vi "Camber controller May 17 2016.vi"() -> ()   [LabVIEW 2014]
uses:
  <vilib>/Instr/_visa.llb/VISA Configure Serial Port (Instr).vi
  Environmental Chamber LabVIEW and Instruments/Drivers and Software/Keithley 2100 Series/Public/Configure/Configure 2 Wire Resistance.vi
  <vilib>/Utility/file.llb/Write To Spreadsheet File (string).vi
  <vilib>/Utility/file.llb/Read From Spreadsheet File (string).vi
  Environmental Chamber LabVIEW and Instruments/Drivers and Software/keithley_6430/Keithley 6430/Public/Data/Read (Single Point).vi
  Environmental Chamber LabVIEW and Instruments/Drivers and Software/LabVIEW 8.2 Drivers/keithley_24xx/Keithley 24XX/Public/Data/Read (Single Point).vi
  Environmental Chamber LabVIEW and Instruments/Drivers and Software/keithley_24xx/Keithley 24XX/Keithley 24XX.lvlib
  Environmental Chamber LabVIEW and Instruments/Drivers and Software/keithley_6430/Keithley 6430/Keithley 6430.lvlib
  Environmental Chamber LabVIEW and Instruments/Drivers and Software/Keithley 2100 Series/Keithley 2100 Series.lvlib
panel:
  out "J-KEM temp chart":dbl(graph)
  out "Elapsed time (min)":dbl
  out "State date/time":string caption="Start time"
  out "Temp (C)":dbl
  in  "Tare elapsed time":bool
  in  "Stop program when sequence ends":bool=TRUE
  out "K-2100 (Ohm)":cluster{"Measurement":dbl}(graph)
  out "pressure chart":cluster{"pressure":dbl}(graph)
  out "K-6430 (Ohm)":cluster{"Measurement":dbl}(graph)
  out "K-2420 (Ohm)":cluster{"Resistance":sgl}(graph)
  in  "Data saving options":T1={"Save during sequence only"=TRUE, "Save now"=FALSE, "Delay between data points (s)"=0.0, "Experiment Notes"="", "Currently saving data"=FALSE, "Data file save path"=path ""} {"Delay between data points (s)" min=0.0 max=30.0 format="%#_13g"}
  in  "Set pressure parameters":T2={"valve % open"=100.0, "Desired pressure"=0.0, "Vapor sccm"=0.0, "Gas sccm"=0.0, "Valve"=enum."% Open", "Pressure Mode"=enum."Abs. pressure", "analyte partial pressure"=100.0} {"analyte partial pressure" min=0.0 max=100.0 step=5.0; "Gas sccm" min=0 max=200 step=5; "Vapor sccm" min=0 max=200 step=5; "Desired pressure" min=0.0 max=760.0 step=5.0; "valve % open" min=0.0 max=100.0 step=5.0 format="%#_2f"}
  out "Actual":T3 {"actual gas flow" format="%#_3g"; "Actual vapor flow" format="%#_3g"; "actual pressure" format="%#_3g"; "Valve position (%)" format="%#_2f"}
  out "Arduino QCM freq":T4 {"QCM1" format="%#_8g"; "QCM2" format="%#_8g"; "QCM3" format="%#_8g"; "QCM4" format="%#_8g"; "QCM5" format="%#_8g"}
  out "Arduino QCM plots":T5
  in  "Sample names":T6={"QCM1"="aQCM2", "QCM2"="aQCM2", "QCM3"="aQCM3", "QCM4"="aQCM4", "QCM5"="aQCM5", "QCM6"="aQCM6", "SRS"="sample_SRS", "K-2420"="Keithley2420", "K-6430"="Keithley6430", "K-2100"="Keithley6430"}
  out "Sequence\npreview":cluster{dbl[], dbl[]}[](graph)
  in  "Gate time":u16(ring)=1 items=["0.1 seconds", "1.0 seconds", "10.0 seconds"]
  out "MHz":dbl format="%.8f"
  out "QCM plot":T7(graph)
  in  "User-defined\nsequence":string[][](table) caption="Create sequence"
  out "Sequence end time":string
  in  "Run Sequence":bool
  in  "Import sequence file":bool
  in  "Save sequence":bool
  in  "Clear sequence":bool
  in  "Turbo pump\nauto on":bool=TRUE caption="Turbo pump auto on"
  in  "Stop":bool
  in  "Clear all charts":bool
  out "appended array":dbl[](array[numeric]) caption="atm\nTorr"
  in  "rapidox O2 Sensor":bool
  in  "setnag O2 Pump":bool
  in  "Baud Rate 2":i32(ring)=2 items=["2400", "4800", "9600", "19200", "38400", "57600", "115200"]
  in  "Com Port":i32(ring) items=["Com 1", "Com 2", "Com 3", "Com 4", "Com 5", "Com 6", "COM 7", "COM 8", "COM 9", "COM 10", "COM 11", "COM 12", "com 13", "COM 14"]
  in  "Com Port 2":i32(ring) items=["Com 1", "Com 2", "Com 3", "Com 4", "Com 5", "Com 6", "COM 7", "COM 8", "COM 9", "COM 10", "COM 11", "COM 12", "com 13", "COM 14"]
  out "Waveform Chart":cluster{dbl}(graph)
  out "O2 Concentration (PPM)":dbl
  out "Waveform Chart 6":cluster{dbl}(graph)
  # "Pressure Control"
  # "Gas Sequence"
  # "SRS QCM"
  # "Currently Unused"
  # "100%"
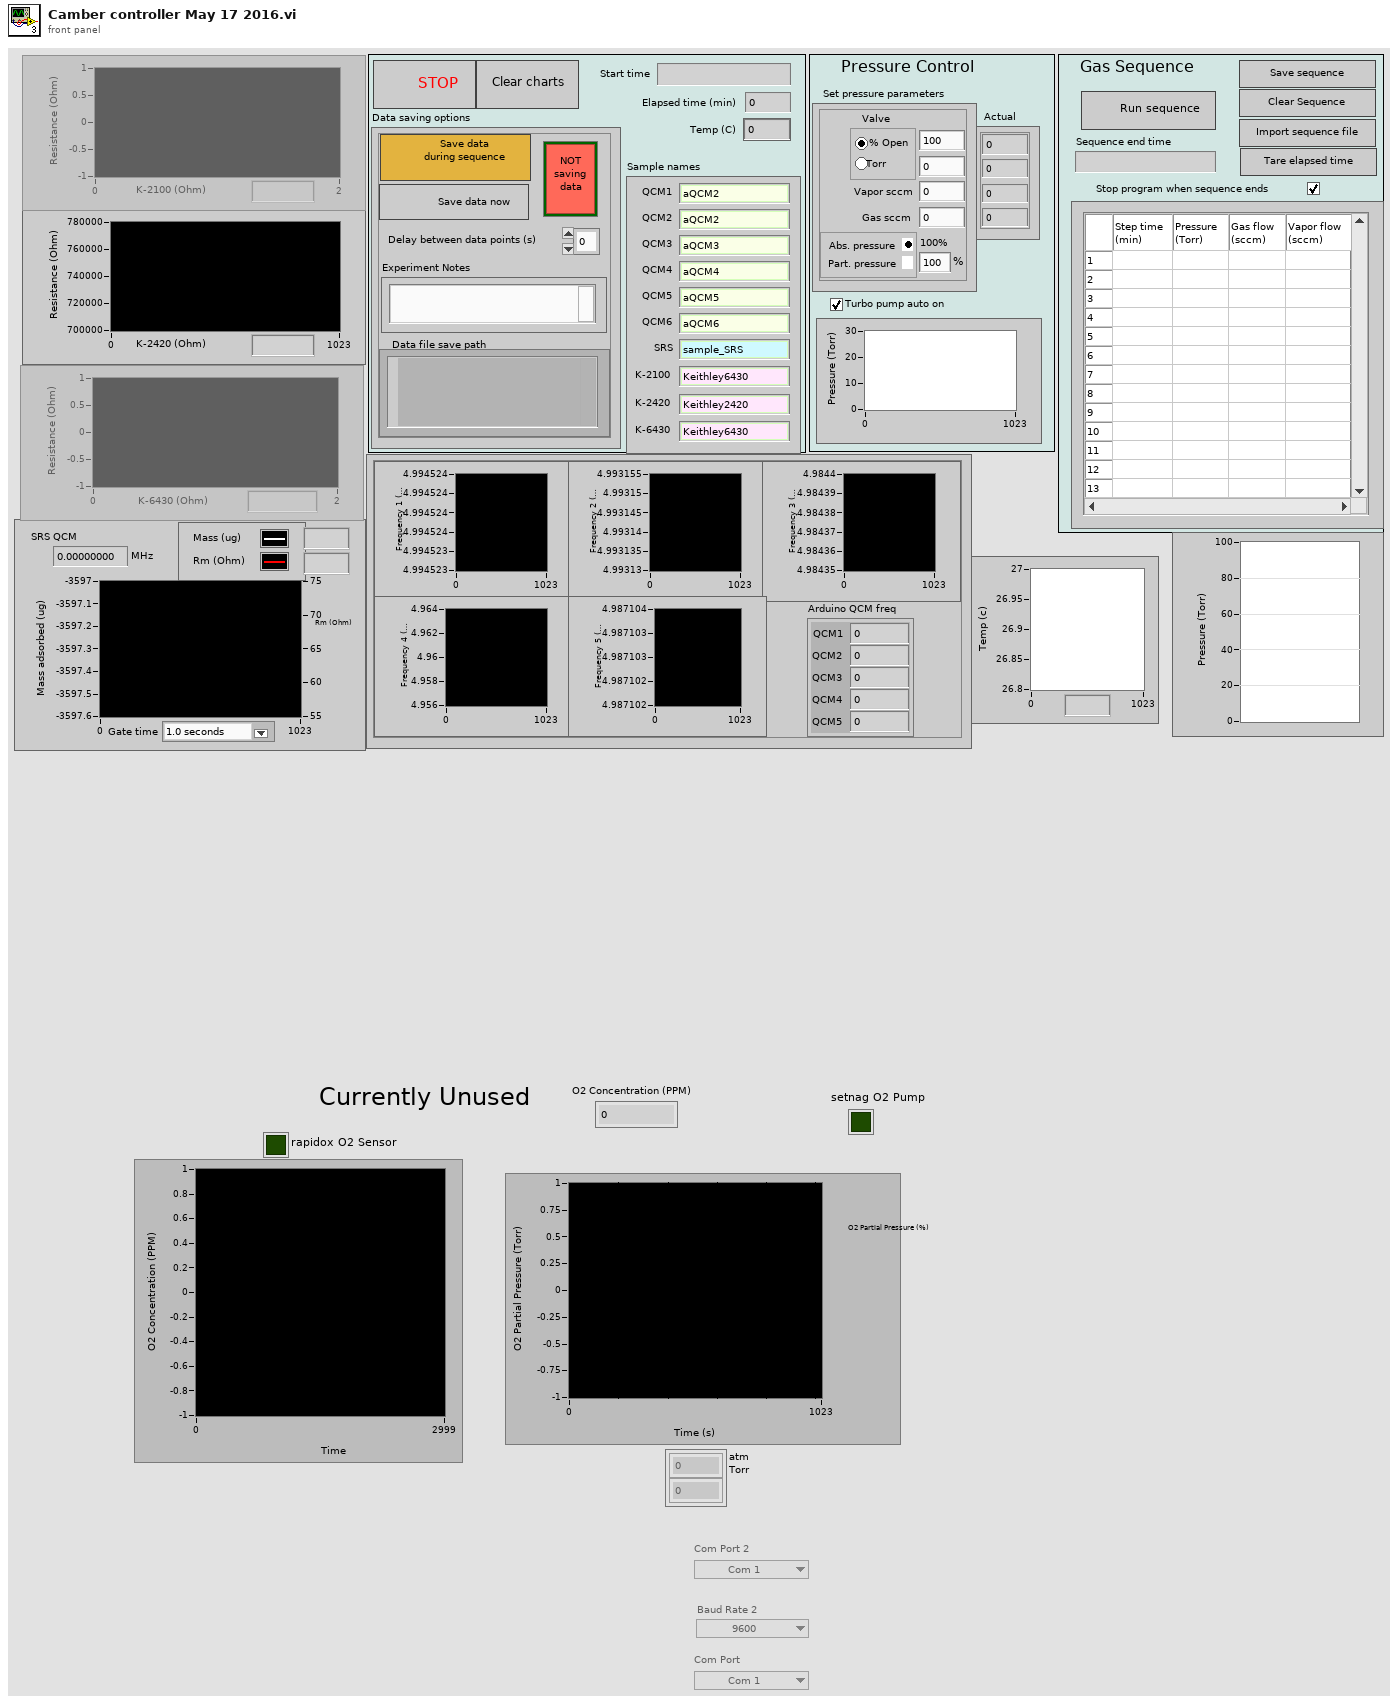
[diagram p1: front panel]
types:
  T1 = cluster{"Save during sequence only":bool, "Save now":bool, "Delay between data points (s)":dbl, "Experiment Notes":string, "Currently saving data":bool, "Data file save path":path}
  T2 = cluster{"valve % open":dbl, "Desired pressure":dbl, "Vapor sccm":sgl, "Gas sccm":sgl, "Valve":enum32{"% Open", "Torr "}, "Pressure Mode":enum32{"Abs. pressure", " Part. pressure"}, "analyte partial pressure":dbl}
  T3 = cluster{"Valve position (%)":dbl, "actual pressure":dbl, "Actual vapor flow":dbl, "actual gas flow":dbl}
  T4 = cluster{"QCM1":dbl, "QCM2":dbl, "QCM3":dbl, "QCM4":dbl, "QCM5":dbl}
  T5 = cluster{"arduino qcm 1":dbl, "arduino qcm 2":dbl, "arduino qcm 3":dbl, "arduino qcm 4":dbl, "arduino qcm 5":dbl}
  T6 = cluster{"QCM1":string, "QCM2":string, "QCM3":string, "QCM4":string, "QCM5":string, "QCM6":string, "SRS":string, "K-2420":string, "K-6430":string, "K-2100":string}
  T7 = cluster{"Numeric Control":dbl, "Resistance out":dbl}
  T8 = cluster{"Arduino 1":refnum<visa-resource-name>, "Arduino 2":refnum<visa-resource-name>, "Arduino 3":refnum<visa-resource-name>, "Arduino 4":refnum<visa-resource-name>, "Arduino 5":refnum<visa-resource-name>}
  T9 = enum16{"open", "open or create", "create or replace", "create", "open (read only)"}
  T10 = enum8{"Enabled", "Disabled", "Disabled and Grayed Out"}
  T11 = enum16{"no parity", "odd parity", "even parity", "mark parity", "space parity"}
  T12 = cluster{"task out":refnum<k21>, "error out":errorcluster, "task out":refnum<k21>, "error out":errorcluster, "task out":refnum<k21>, "error out":errorcluster, "VISA resource name":refnum<visa-resource-name>, "error out":errorcluster}
  T13 = cluster{"task out":refnum<k21>, "error out":errorcluster, "task out":refnum<k21>, "error out":errorcluster, "task out":refnum<k21>, "error out":errorcluster, "VISA resource name out":refnum<visa-resource-name>, "error out":errorcluster}
  T14 = cluster{bool, "VISA resource name":refnum<visa-resource-name>, "error out":errorcluster}
  T15 = cluster{bool, "VISA resource name out":refnum<visa-resource-name>, "error out":errorcluster}
  T16 = cluster{"VISA resource name out":refnum<visa-resource-name>, "error out":errorcluster, "VISA resource name out":refnum<visa-resource-name>, "error out":errorcluster, "VISA resource name out":refnum<visa-resource-name>, "error out":errorcluster, "VISA resource name out":refnum<visa-resource-name>, "error out":errorcluster, "VISA resource name out":refnum<visa-resource-name>, "error out":errorcluster}
  T17 = cluster{"f":dbl, "f":dbl, "f":dbl, "f":dbl, "f":dbl}
  T18 = cluster{"String":string, "String":string, "String":string}
  T19 = cluster{"Boolean":bool, "VISA resource name out":refnum<visa-resource-name>, "error out":errorcluster}
  T20 = cluster{bool, "VISA out":refnum<visa-resource-name>, "error out":errorcluster}
  T21 = cluster{"Boolean":bool, "VISA out":refnum<visa-resource-name>, "error out":errorcluster}
  T22 = cluster{"Numeric Control":dbl, "Cluster":cluster{"Numeric Control":dbl}, "String":string, "error out":errorcluster}
  T23 = cluster{bool, "Com Port":i32, "Numeric Control out":dbl}
  T24 = cluster{"String data out":string, string, string, string}
  T25 = cluster{"User-defined\nsequence":refnum<vi>, "Sequence end time":refnum<vi>, "Run Sequence":refnum<vi>}
  T26 = cluster{"Present (s)":dbl, "Run Sequence":bool, "Set pressure parameters":cluster{"valve % open":dbl, "Desired pressure":dbl, "Vapor sccm":sgl, "Gas sccm":sgl, "Valve":enum32{"% Open", "Torr "}, "Pressure Mode":enum32{"Abs. pressure", " Part. pressure"}, "analyte partial pressure":dbl}, "sequence end time":timestamp}
  T27 = cluster{bool, "Turbo pump\nauto on":bool, "current  step # out":i32, cluster{"Present (s)":dbl, "Run Sequence":bool, "Set pressure parameters":cluster{"valve % open":dbl, "Desired pressure":dbl, "Vapor sccm":sgl, "Gas sccm":sgl, "Valve":enum32{"% Open", "Torr "}, "Pressure Mode":enum32{"Abs. pressure", " Part. pressure"}, "analyte partial pressure":dbl}, "sequence end time":timestamp}}
  T28 = cluster{"pressure":string, "RH":string, "gas flow":string, "vapor flow":string}
  T29 = cluster{"Valve position (%)":dbl, "pressure":dbl, "vapor flow":dbl, "gas flow":dbl}
  T30 = cluster{"sequence on?":bool, "current  step # out":i32, "sequence end time":timestamp}
  T31 = cluster{"task out":refnum<k21>, "error out":errorcluster, "task out":refnum<k21>, "error out":errorcluster, "task out":refnum<k21>, "error out":errorcluster, "VISA Refnum out":refnum<visa-resource-name>, "error out":errorcluster}
  T32 = cluster{"VISA Refnum out":refnum<visa-resource-name>, "error out":errorcluster, "VISA Refnum out":refnum<visa-resource-name>, "error out":errorcluster, "VISA Refnum out":refnum<visa-resource-name>, "error out":errorcluster, "VISA Refnum out":refnum<visa-resource-name>, "error out":errorcluster, "VISA Refnum out":refnum<visa-resource-name>, "error out":errorcluster}
  T33 = cluster{"f":string, "f":string, "f":string, "f":string, "f":string}
  T34 = cluster{"f":dbl, "f":dbl, "f":dbl, "f":dbl, "f":dbl}[]
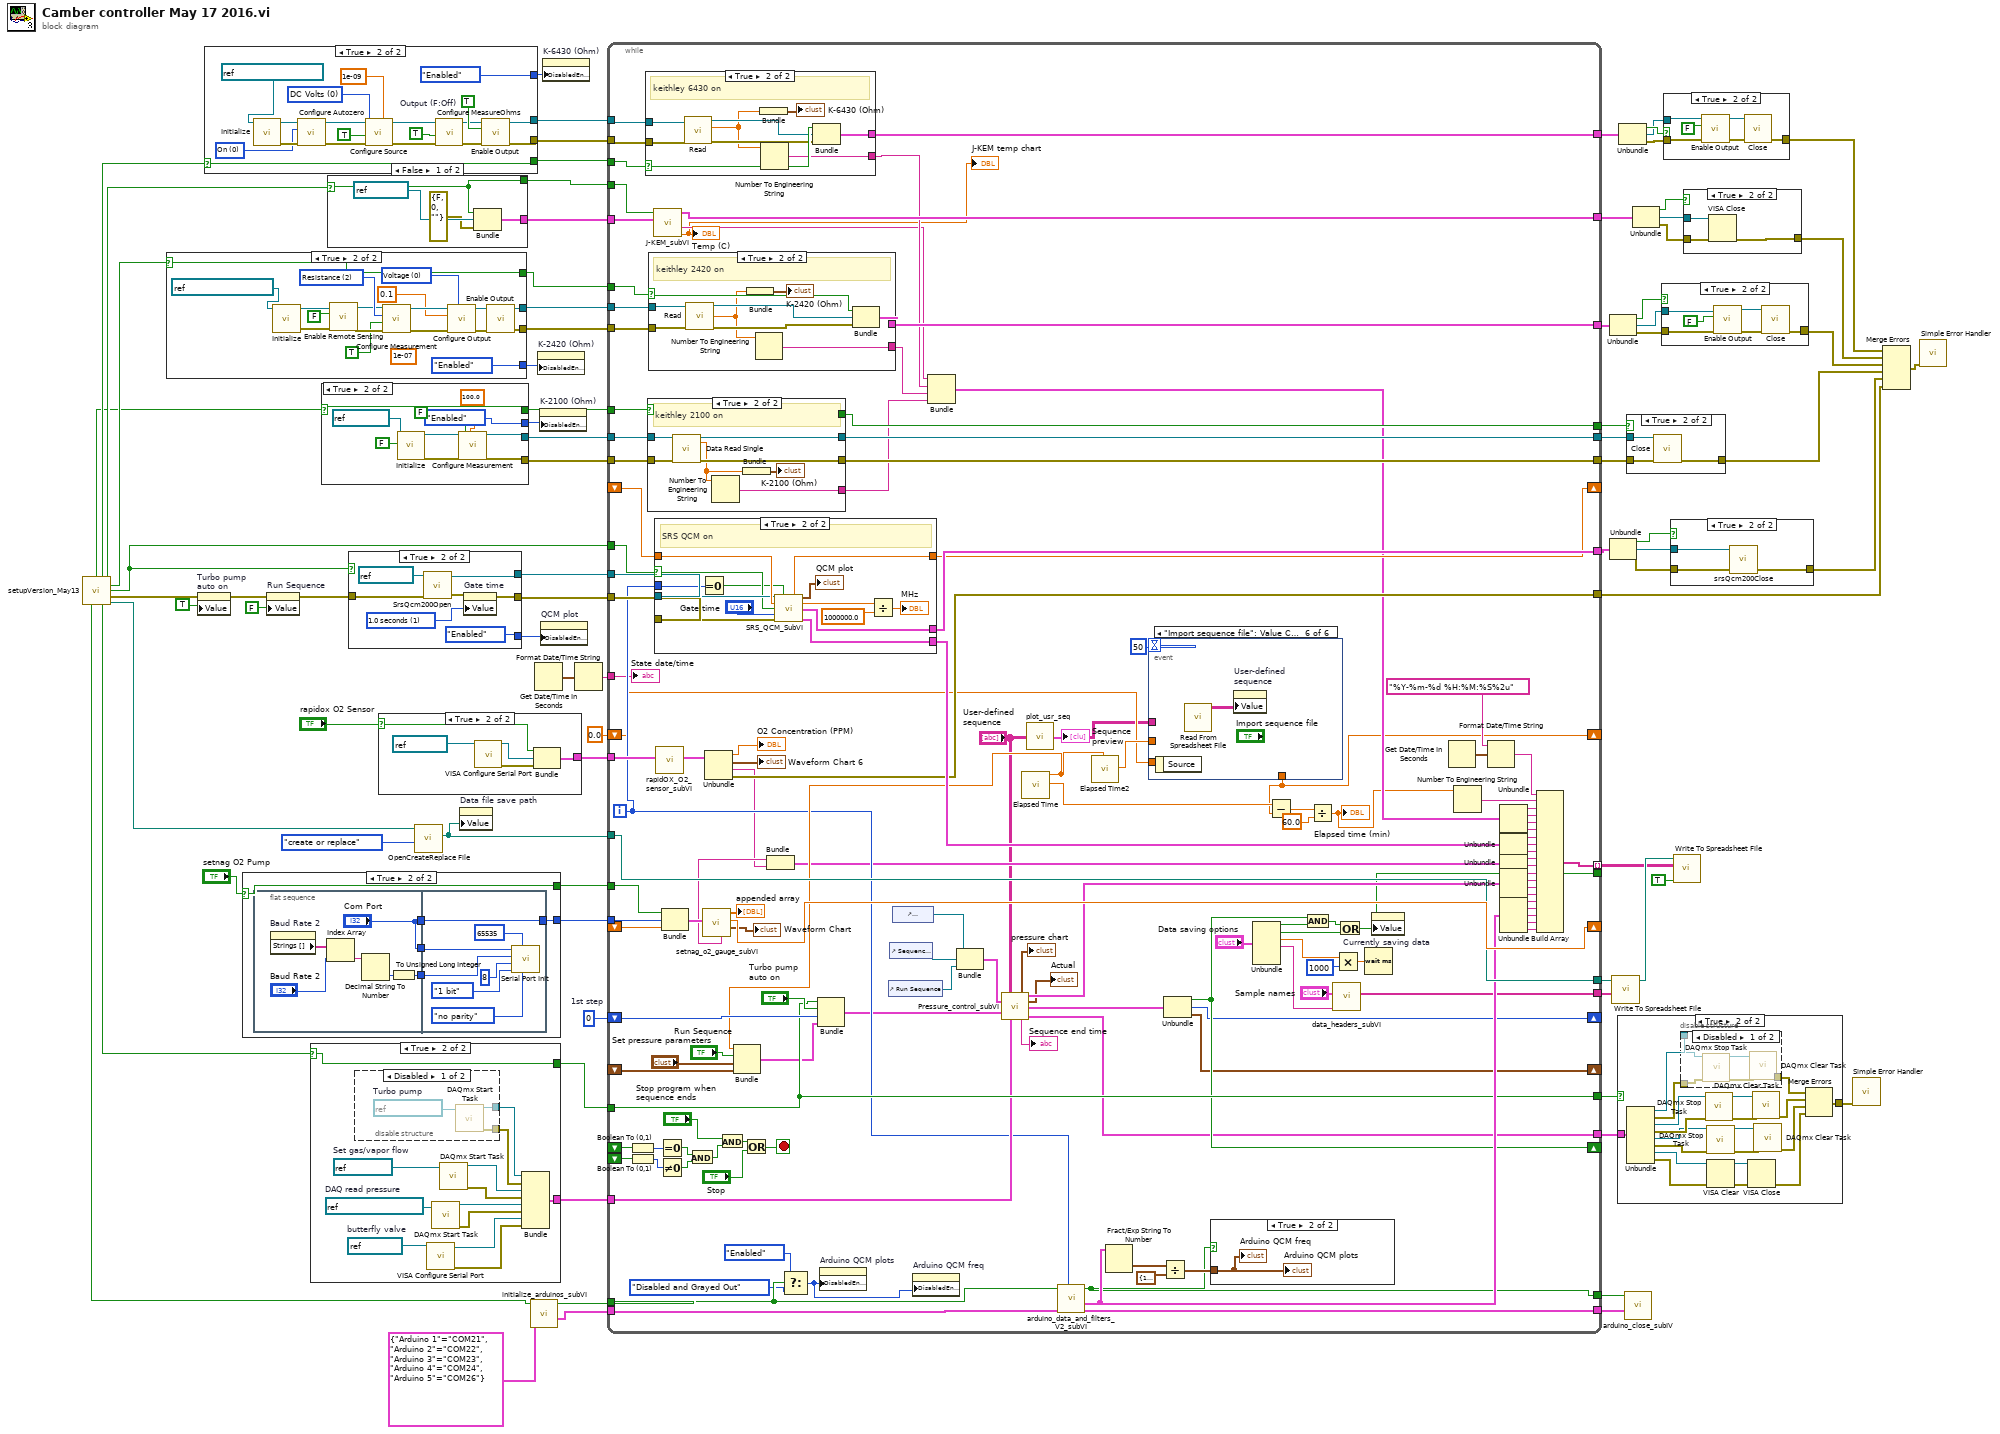
[diagram p0: block diagram]
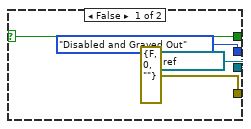
[diagram p3: hidden frame]
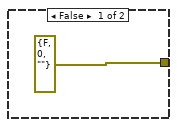
[diagram p4: hidden frame]
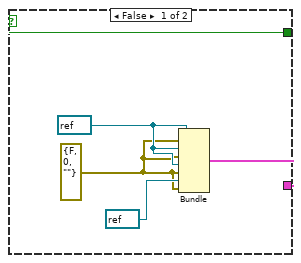
[diagram p6: hidden frame]
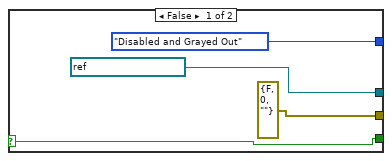
[diagram p9: hidden frame]
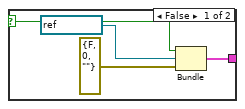
[diagram p10: hidden frame]
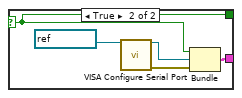
[diagram p12: hidden frame]
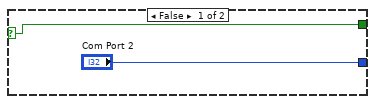
[diagram p13: hidden frame]
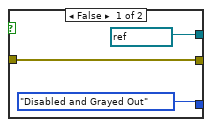
[diagram p15: hidden frame]
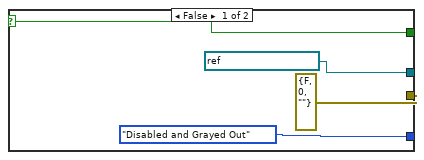
[diagram p17: hidden frame]
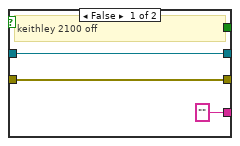
[diagram p19: hidden frame]
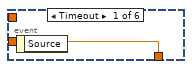
[diagram p20: hidden frame]
diagram:
  w42 = 0  # 1st step
  n1 = call "setupVersion_May13.vi"() -> ("Keithley 2100 out"=w11:bool, "Keithley 6431"=w35:bool, "J-KEM2"=w34:bool, "Keithley 2421"=w23:bool, "SRS QCM 2"=w37:bool, "error IO"=w1:errorcluster, "Arduino2"=w28:bool, "Pressure control 2"=w36:bool, "Save file path 2"=w2:path)  [unwired: 7 in]
  n2 = case shown="True" w23 {
    selector: w23 -> [w83 w87]
    tunnel: [refnum<visa-resource-name> "GPIB1::24::INSTR" ("VISA resource name") w96] -> w80
    tunnel: [errorcluster {"status"=FALSE, "code"=0, "source"=""} ("error out") w91] -> w79
    tunnel: [T10."Disabled and Grayed Out" ("Disabled") T10."Enabled" ("Disabled")] -> w32
    tunnel: [w83 w87] -> w22
    frame False {
    }
    frame True {
      (unwired) 1e-07 ("Manual Range (1.0)")
      w98 = u16 0 items=["Voltage", "Current"] ("Source Mode  (0: Voltage)")
      w103 = u16 2 items=["Volts", "Current", "Resistance"] ("Function (0: Volts)")
      n3 = call "Initialize.vi"("VISA resource name"=refnum<visa-resource-name> "GPIB1::24::INSTR") -> ("error out"=w92:errorcluster, "VISA resource name out"=w95:refnum<visa-resource-name>)  [unwired: 9 in]
      n4 = call "Enable Remote Sensing.vi"("error in (no error)"=w92, "Enable Remote Sensing (T: Enable)"=FALSE ("4-wire?"), "VISA resource name"=w95) -> ("error out"=w93:errorcluster, "VISA resource name out"=w94:refnum<visa-resource-name>)  [unwired: 7 in]
      n5 = call "Configure Measurement.vi"("error in (no error)"=w93, "Enable Auto Range (T:Enable)"=TRUE, "Function (0: Volts)"=w103, "VISA resource name"=w94) -> ("error out"=w102:errorcluster, "VISA resource name out"=w101:refnum<visa-resource-name>)  [unwired: 6 in]
      n6 = call "Configure Output.vi"("Source Mode  (0: Voltage)"=w98, "error in (no error)"=w102, "Output Level (0)"=0.1 ("Applied Voltage (V)"), "VISA resource name"=w101) -> ("error out"=w100:errorcluster, "VISA resource name out"=w99:refnum<visa-resource-name>)  [unwired: 6 in]
      n7 = call "Enable Output.vi"("error in (no error)"=w100, "VISA resource name"=w99) -> ("error out"=w91:errorcluster, "VISA resource name out"=w96:refnum<visa-resource-name>)  [unwired: 8 in]
    }
  }
  n8 = property on="Turbo pump\nauto on" class="Bool (strict)"(error in=w1, "Value"=TRUE ("Turbo\npump")) -> (error out=w38:errorcluster)  [unwired: 1 in, 1 out]
  n9 = case shown="True" w35 {
    selector: w35 -> [w105 w109]
    tunnel: [refnum<visa-resource-name> "GPIB0::29::INSTR" ("VISA resource name") w122] -> w49
    tunnel: [errorcluster {"status"=FALSE, "code"=0, "source"=""} ("error out") w123] -> w48
    tunnel: [T10."Disabled and Grayed Out" ("Disabled") T10."Enabled" ("Disabled")] -> w31
    tunnel: [w105 w109] -> w21
    frame False {
    }
    frame True {
      w111 = u16 0 items=["DC Volts", "DC Current"] ("Source Function (0: DC Volts)")
      w118 = u16 0 items=["On", "Off", "Once"] ("Autozero  (0: On)")
      w126 = TRUE  # Output (F:Off)
      n10 = call "Initialize.vi"("VISA resource name"=refnum<visa-resource-name> "GPIB0::30::INSTR") -> ("error out"=w119:errorcluster, "VISA resource name out"=w120:refnum<visa-resource-name>)  [unwired: 4 in, 5 out]
      n11 = call "Configure Autozero.vi"("error in (no error)"=w119, "Autozero  (0: On)"=w118, "VISA resource name"=w120) -> ("error out"=w114:errorcluster, "VISA resource name out"=w116:refnum<visa-resource-name>)  [unwired: 7 in]
      n12 = call "Configure Source.vi"("I-Source Level [A]"=1e-09, "error in (no error)"=w114, "Auto Range (T:Enable)"=TRUE, "Source Function (0: DC Volts)"=w111, "VISA resource name"=w116) -> ("error out"=w113:errorcluster, "VISA resource name out"=w115:refnum<visa-resource-name>)  [unwired: 5 in]
      n13 = call "Configure MeasureOhms.vi"("error in (no error)"=w113, "Auto Range (T:Enable)"=TRUE, "VISA resource name"=w115) -> ("error out"=w127:errorcluster, "VISA resource name out"=w125:refnum<visa-resource-name>)  [unwired: 3 in, 4 out]
      n14 = call "Enable Output.vi"("error in (no error)"=w127, "Enable Output (F:Off)"=w126, "VISA resource name"=w125) -> ("error out"=w123:errorcluster, "VISA resource name out"=w122:refnum<visa-resource-name>)  [unwired: 7 out]
    }
  }
  n15 = case shown="True" "setnag O2 Pump" {
    selector: "setnag O2 Pump" -> [w128 w130]
    tunnel: ["Com Port 2" w131] -> w76
    tunnel: [w128 w130] -> w8
    frame False {
    }
    frame True {
      n16 = flat-sequence {
        tunnel: ["Com Port"] -> w134
        tunnel: [w136] -> w133
        tunnel: ["Com Port"] -> w132
        tunnel: w134 -> [w142]
        tunnel: w133 -> [w141]
        tunnel: w132 -> [w143]
        tunnel: [w143] -> w131
        frame #0 {
          n17 = property on="Baud Rate 2" class="Ring (strict)"() -> ("Strings []"=w138:string[])  [unwired: 2 in, 2 out]
          n18 = Index Array(array=w138, index="Baud Rate 2") -> (element=w139:string)
          n19 = Decimal String To Number(string=w139) -> (number=w137:i32)  [unwired: 2 in, 1 out]
          n20 = To Unsigned Long Integer(number=w137) -> (unsigned 32bit integer=w136:u32)
        }
        frame #1 {
          n21 = call <vilib>:"Serial Port Init.vi"("parity"=T11."no parity", "buffer size"=u16 65535, "stop bits"=enum16{"1 bit", "1.5 bits", "2 bits"}."1 bit", "data bits"=u16 8, "baud rate"=w141, "port number"=w142) -> ()  [unwired: 1 in, 1 out]
        }
      }
    }
  }
  n22 = property on="Run Sequence" class="Bool (strict)"(error in=w38, "Value"=FALSE ("Run Sequence")) -> (error out=w40:errorcluster)  [unwired: 1 in, 1 out]
  n23 = case shown="True" w36 {
    selector: w36 -> [w148 w153]
    tunnel: [w149 w155] -> w43
    tunnel: [w148 w153] -> w20
    frame False {
      w151 = refnum<k21> refnum ("task out")
      w150 = errorcluster {"status"=FALSE, "code"=0, "source"=""} ("error out")
      n24 = Bundle("task out"=w151, "error out"=w150, "task out"=w151, "error out"=w150, "task out"=w151, "error out"=w150, "VISA resource name"=refnum<visa-resource-name> refnum, "error out"=w150) -> (w149:T12)  [unwired: 1 in]
    }
    frame True {
      w163 = refnum<visa-resource-name> "COM5"  # butterfly valve
      w164 = refnum<k21> "Setflow"  # Set gas/vapor flow
      w165 = refnum<k21> "AllDaqReadings"  # DAQ read pressure
      n25 = disable-structure shown="Disabled" {
        disable-tunnel: [w167 _] -> w162
        disable-tunnel: [w166 _] -> w161
        frame Disabled {
          w168 = refnum<k21> "TurboON"  # Turbo pump
          n26 = call <vilib>:"DAQmx Start Task.vi"("task/channels in"=w168) -> ("task out"=w167:refnum<k21>, "error out"=w166:errorcluster)  [unwired: 13 in]
        }
        frame Enabled {
        }
      }
      n27 = call-poly "VISA Configure Serial Port"("VISA resource name"=w163) -> ("VISA resource name out"=w156:refnum<visa-resource-name>, "error out"=w154:errorcluster)  [unwired: 13 in]
      n28 = call <vilib>:"DAQmx Start Task.vi"("task/channels in"=w165) -> ("task out"=w158:refnum<k21>, "error out"=w157:errorcluster)  [unwired: 13 in]
      n29 = call <vilib>:"DAQmx Start Task.vi"("task/channels in"=w164) -> ("task out"=w160:refnum<k21>, "error out"=w159:errorcluster)  [unwired: 13 in]
      n30 = Bundle("task out"=w162, "error out"=w161, "task out"=w160, "error out"=w159, "task out"=w158, "error out"=w157, "VISA resource name out"=w156, "error out"=w154) -> (w155:T13)  [unwired: 1 in]
    }
  }
  n31 = case shown="True" w11 {
    selector: w11 -> [w170 w176]
    tunnel: [refnum<visa-resource-name> "K-2100" ("VISA resource name out") w179] -> w18
    tunnel: [errorcluster {"status"=FALSE, "code"=0, "source"=""} ("error out") w178] -> w17
    tunnel: [w170 w176] -> w16
    tunnel: [T10."Disabled and Grayed Out" ("Disabled") T10."Enabled" ("Disabled")] -> w10
    frame False {
    }
    frame True {
      n32 = call "Initialize.vi"("VISA resource name"=refnum<visa-resource-name> "K-2100", "Reset? (T: Reset)"=FALSE) -> ("VISA resource name out"=w180:refnum<visa-resource-name>, "error out"=w177:errorcluster)  [unwired: 16 in]
      n33 = call-poly "Configure Measurement.vi"("VISA resource name"=w180, "error in (no error)"=w177, "Auto Range? (T: Auto)"=FALSE, "Custom Range (100 Ohm)"=100.0 ("Temp (C) 2")) -> ("VISA resource name out"=w179:refnum<visa-resource-name>, "error out"=w178:errorcluster)  [unwired: 14 in]
    }
  }
  n34 = case shown="False" w34 {
    selector: w34 -> [w183 w188]
    tunnel: [w184 w189] -> w65
    tunnel: [w183 w188] -> w59
    frame False {
      n35 = Bundle(w183, "VISA resource name"=refnum<visa-resource-name> "COM3", "error out"=errorcluster {"status"=FALSE, "code"=0, "source"=""}) -> (w184:T14)  [unwired: 1 in]
    }
    frame True {
      n36 = call-poly "VISA Configure Serial Port"("VISA resource name"=refnum<visa-resource-name> "COM3") -> ("VISA resource name out"=w190:refnum<visa-resource-name>, "error out"=w187:errorcluster)  [unwired: 13 in]
      n37 = Bundle(w188, "VISA resource name out"=w190, "error out"=w187) -> (w189:T15)  [unwired: 1 in]
    }
  }
  n38 = case shown="True" w37 {
    tunnel: [refnum<visa-resource-name> "COM6" ("VISA in") w198] -> w78
    tunnel: [w193 w195] -> w77
    tunnel: w40 -> [w193 w200]
    tunnel: [T10."Disabled and Grayed Out" ("Disabled") T10."Enabled" ("Disabled")] -> w33
    frame False {
    }
    frame True {
      w197 = u16 1 items=["0.1 seconds", "1.0 seconds", "10.0 seconds"] ("Gate time")
      n39 = call "SrsQcm200Open.vi"("error in"=w200, "VISA in"=refnum<visa-resource-name> "COM6") -> ("error out"=w196:errorcluster, "VISA out"=w198:refnum<visa-resource-name>)  [unwired: 3 in]
      n40 = property on="Gate time" class="Ring (strict)"(error in=w196, "Value"=w197) -> (error out=w195:errorcluster)  [unwired: 1 in, 1 out]
    }
  }
  n41 = case shown="True" "rapidox O2 Sensor" {
    selector: "rapidox O2 Sensor" -> [w202 w207]
    tunnel: [w203 w208] -> w55
    frame False {
      n42 = Bundle(w202, "VISA resource name"=refnum<visa-resource-name> "COM7", "error out"=errorcluster {"status"=FALSE, "code"=0, "source"=""}) -> (w203:T14)  [unwired: 1 in]
    }
    frame True {
      n43 = call-poly "VISA Configure Serial Port"("VISA resource name"=refnum<visa-resource-name> "COM7") -> ("VISA resource name out"=w209:refnum<visa-resource-name>, "error out"=w206:errorcluster)  [unwired: 13 in]
      n44 = Bundle(w207, "VISA resource name out"=w209, "error out"=w206) -> (w208:T15)  [unwired: 1 in]
    }
  }
  n45 = call "OpenCreateReplace File.vi"("function (open:0)"=T9."create or replace", "file path"=w2) -> ("new file path"=w19:path)  [unwired: 6 in, 3 out]
  n46 = property on="Data file save path" class="Path"("Value"=w19) -> ()  [unwired: 2 in, 2 out]
  n47 = call "initialize_arduinos_subVI.vi"("arduino 1-6 addresses"=T8 {"Arduino 1"="COM21", "Arduino 2"="COM22", "Arduino 3"="COM23", "Arduino 4"="COM24", "Arduino 5"="COM26"}, "arduinos on?"=w28) -> ("arduino addresses/errors"=w3:T16, "arduinos on/off"=w29:bool)  [unwired: 8 in]
  n48 = Get Date/Time In Seconds() -> (seconds since 1Jan1904=w82:timestamp)
  n49 = property on="K-2420 (Ohm)" class="WFChart (strict)"("DisabledEnum"=w32) -> ()  [unwired: 2 in, 2 out]
  n50 = property on="K-2100 (Ohm)" class="WFChart (strict)"("DisabledEnum"=w10) -> ()  [unwired: 2 in, 2 out]
  n51 = property on="QCM plot" class="WFChart (strict)"("DisabledEnum"=w33) -> ()  [unwired: 2 in, 2 out]
  n52 = property on="K-6430 (Ohm)" class="WFChart (strict)"("DisabledEnum"=w31) -> ()  [unwired: 2 in, 2 out]
  n53 = Format Date/Time String(seconds (now)=w82) -> (date/time string=w7:string)  [unwired: 2 in]
  n54 = while {
    shift-right: [w346] -> _
    shift-left: _ -> [w240]
    tunnel: [w329] -> w30 mode=indexing if=w274
    tunnel: w22 -> [w335]
    tunnel: w80 -> [w345]
    tunnel: w79 -> [w344]
    tunnel: w78 -> [w343]
    tunnel: w77 -> [w342]
    tunnel: w37 -> [w341]
    tunnel: w8 -> [w242]
    tunnel: w76 -> [w243]
    tunnel: [w340] -> w73
    tunnel: [w339] -> w69
    tunnel: w65 -> [w338]
    tunnel: [w337] -> w64
    tunnel: w59 -> [w336]
    tunnel: w55 -> [w257]
    tunnel: [w253] -> w5
    tunnel: [w334] -> w54
    tunnel: w19 -> [w334]
    shift-right: [w327] -> _
    shift-left: _ -> [w328]
    tunnel: w49 -> [w333]
    tunnel: w48 -> [w332]
    tunnel: [w331] -> w47
    tunnel: w20 -> [w292]
    tunnel: [w292] -> w44
    tunnel: w43 -> [w290]
    shift-right: [w215] -> _
    shift-left: w42 -> [w294]
    tunnel: [w274] -> _
    shift-right: [w214] -> _
    shift-left: _ -> [w302]
    tunnel: w29 -> [w252]
    tunnel: w3 -> [w320]
    tunnel: [w248] -> w26
    tunnel: [w319] -> w27
    tunnel: [w311] -> w25
    tunnel: [w213] -> w24
    tunnel: w21 -> [w303]
    shift-right: [w216] -> _
    shift-left: _ -> [w289]
    shift-left: _ -> [w288]
    tunnel: w18 -> [w272]
    tunnel: w17 -> [w271]
    tunnel: w16 -> [w270]
    tunnel: [w269] -> w15
    tunnel: [w268] -> w14
    tunnel: [w267] -> w13
    shift-right: [w234] -> _
    shift-left: 0.0 ("Elapsed Time (s)") -> [w235]
    tunnel: w7 -> [w225]
    i -> [w244]
    stop <- w278 stop-if-true
    n55 = Boolean To (0,1)(Boolean=w289) -> (0, 1=w287:i16)
    n56 = Boolean To (0,1)(Boolean=w288) -> (0, 1=w286:i16)
    n57 = case "Keithley 6430" shown="True" w303 {
      selector: w303 -> [w376 w386]
      tunnel: w333 -> [w375 w383]
      tunnel: w332 -> [w374 w382]
      tunnel: ["" w385] -> w247
      tunnel: [w373 w384] -> w331
      frame False {
        # "keithley 6430 off"
        n58 = Bundle(w376, "VISA resource name out"=w375, "error out"=w374) -> (w373:T15)  [unwired: 1 in]
      }
      frame True {
        # "keithley 6430 on"
        n59 = call-poly "Read.vi"("error in (no error)"=w382, "VISA resource name"=w383) -> ("error out"=w381:errorcluster, "Measurement"=w379:dbl, "VISA resource name out"=w380:refnum<visa-resource-name>)  [unwired: 1 in, 6 out]
        n60 = Bundle("Measurement"=w379) -> (→"K-6430 (Ohm)":cluster{"Measurement":dbl})  [unwired: 1 in]
        n61 = Number To Engineering String(4:w379) -> (0:w385:string)  [unwired: 3 in]
        n62 = Bundle(w386, "VISA resource name out"=w380, "error out"=w381) -> (w384:T15)  [unwired: 1 in]
      }
    }
    n63 = case shown="True" w270 {
      selector: w270 -> [w349 w353]
      tunnel: [w350 w360] -> w268
      tunnel: [w351 w359] -> w267
      tunnel: w272 -> [w350 w358]
      tunnel: w271 -> [w351 w357]
      tunnel: ["" w355] -> w245
      tunnel: [w349 w353] -> w269
      frame False {
        # "keithley 2100 off"
      }
      frame True {
        # "keithley 2100 on"
        n64 = call "Data Read Single.vi"("VISA resource name"=w358, "error in (no error)"=w357) -> ("VISA resource name out"=w360:refnum<visa-resource-name>, "Measurement"=w356:dbl, "error out"=w359:errorcluster)  [unwired: 15 in]
        n65 = Number To Engineering String ("elapsed time (min)")(4:w356) -> (0:w355:string)  [unwired: 3 in]
        n66 = Bundle("Measurement"=w356) -> (→"K-2100 (Ohm)":cluster{"Measurement":dbl})  [unwired: 1 in]
      }
    }
    n67 = case "Keithley 2420" shown="True" w335 {
      selector: w335 -> [w390 w398]
      tunnel: w345 -> [w389 w393]
      tunnel: w344 -> [w388 w392]
      tunnel: [w387 w396] -> w340
      tunnel: ["" w395] -> w246
      frame False {
        # "keithley 2420 off"
        n68 = Bundle(w390, "VISA resource name out"=w389, "error out"=w388) -> (w387:T15)  [unwired: 1 in]
      }
      frame True {
        # "keithley 2420 on"
        n69 = call-poly "Read.vi"("VISA resource name"=w393, "error in (no error)"=w392) -> ("VISA resource name out"=w399:refnum<visa-resource-name>, "Resistance"=w394:sgl, "error out"=w397:errorcluster)  [unwired: 7 in, 4 out]
        n70 = Bundle("Resistance"=w394) -> (→"K-2420 (Ohm)":cluster{"Resistance":sgl})  [unwired: 1 in]
        n71 = Number To Engineering String(4:w394) -> (0:w395:string)  [unwired: 3 in]
        n72 = Bundle(w398, "VISA resource name out"=w399, "error out"=w397) -> (w396:T15)  [unwired: 1 in]
      }
    }
    n73 = call "J-KEM_subVI.vi"("Address in"=w338, "J-KEM on?"=w336) -> ("Temp (C)"=→"Temp (C)" →"J-KEM temp chart":dbl, "String data out"=w233:string, "Address out"=w337:T19)  [unwired: 6 in, 1 out]
    n74 = case "SRS QCM" shown="True" w341 {
      selector: w341 -> [w403 w414]
      tunnel: w343 -> [w406 w416]
      tunnel: w342 -> [w405 w417]
      tunnel: [w404 w420] -> w339
      tunnel: w328 -> [w401 w419]
      tunnel: [w401 w418] -> w327
      tunnel: [T18 {"String"="", "String"="", "String"=""} ("M,F,MR output cluster") w413] -> w317
      tunnel: w244 -> [_ w407]
      frame False {
        # "SRS QCM off"
        n75 = Bundle(w403, "VISA out"=w406, "error out"=w405) -> (w404:T20)  [unwired: 1 in]
      }
      frame True {
        # "SRS QCM on"
        n76 = Equal To 0?(x=w407) -> (x = 0?=w408:bool)
        n77 = call "SRS_QCM_SubVI.vi"("VISA Refnum in"=w416, "first iteration?"=w408, "Frequency out 3"=w419, "Boolean 2"=w414, "Gate time"="Gate time", "error in (no error)"=w417) -> ("Frequency out 2"=w418:dbl, "Cluster"=→"QCM plot":T7, "Frequency out"=w409:dbl, "Cluster 2"=w420:T21, "M,F,MR output cluster"=w413:T18)  [unwired: 2 in, 3 out]
        n78 = Divide(x=w409, y=1000000.0) -> (x/y=→"MHz":dbl)
      }
    }
    n79 = call "rapidOX_O2_sensor_subVI.vi"("rapid ox info in"=w257) -> ("rapidox info out"=w256:T22)  [unwired: 10 in]
    n80 = Equal To 0?(x=w287) -> (x = 0?=w284:bool)
    n81 = Not Equal To 0?(x=w286) -> (x != 0?=w285:bool)
    n82 = Bundle(w242, "Com Port"=w243, "Numeric Control out"=w240) -> (w241:T23)  [unwired: 1 in]
    n83 = And(x=w284, y=w285) -> (x .and. y?=w277:bool)
    n84 = call "setnag_o2_gauge_subVI.vi"("setnag info in"=w241) -> ("Cluster"=→"Waveform Chart":cluster{"Numeric Control":dbl}, "Numeric Control out"=w346:dbl, "Array"=→"appended array":dbl[], "String"=w224:string)  [unwired: 7 in]
    n85 = Unbundle(w256) -> ("Numeric Control"=→"O2 Concentration (PPM)":dbl, "Cluster"=→"Waveform Chart 6":cluster{"Numeric Control":dbl}, "String"=w223:string, "error out"=w253:errorcluster)
    n86 = And(x="Stop program when sequence ends", y=w277) -> (x .and. y?=w238:bool)
    n87 = Or(x=w238, y="Stop") -> (x .or. y?=w278:bool)
    n88 = Bundle("String"=w224, "String"=w223) -> (w222:cluster{"String":string, "String":string})  [unwired: 1 in]
    n89 = Select(t=T10."Enabled" ("Disabled"), s=w252, f=T10."Disabled and Grayed Out" ("Disabled")) -> (s? t:f=w250:T10)
    n90 = property on="Arduino QCM plots" class="Clust (strict)"("DisabledEnum"=w250) -> ()  [unwired: 2 in, 2 out]
    n91 = control-ref of="Run Sequence"() -> (w296:refnum<vi>)
    n92 = control-ref of="Sequence end time"() -> (w297:refnum<vi>)
    n93 = control-ref of="User-defined\nsequence"() -> (w298:refnum<vi>)
    n94 = property on="Arduino QCM freq" class="Clust (strict)"("DisabledEnum"=w250) -> ()  [unwired: 2 in, 2 out]
    n95 = Bundle("String data out"=w233, w247, w246, w245) -> (w239:T24)  [unwired: 1 in]
    n96 = Bundle("User-defined\nsequence"=w298, "Sequence end time"=w297, "Run Sequence"=w296) -> (w295:T25)  [unwired: 1 in]
    n97 = call "Elapsed Time"() -> ("Present (s)"=w261:dbl, "Elapsed Time (s)"=w259:dbl)  [unwired: 12 in, 6 out]
    n98 = Bundle("Present (s)"=w261, "Run Sequence"="Run Sequence", "Set pressure parameters"="Set pressure parameters", "sequence end time"=w302) -> (w218:T26)  [unwired: 1 in]
    n99 = Bundle(w292, "Turbo pump\nauto on"="Turbo pump\nauto on", "current  step # out"=w294, w218) -> (w217:T27)  [unwired: 1 in]
    n100 = call "Pressure_control_subVI.vi"("User-defined\nsequence"="User-defined\nsequence", "references in"=w295, "pressure controlk / turbo / current step / present sec/run seq/press settings"=w217, "DAQ IDs in"=w290) -> ("pressure"=→"pressure chart":cluster{"pressure":dbl}, "press/RH/gas/vapor"=w308:T28, "pressure params out"=→"Actual":T29, "seq on/end time/current step"=w212:T30, "date/time string"=→"Sequence end time":string, "DAQ IDs out"=w213:T31)  [unwired: 6 in]
    n101 = call "plot_usr_seq.vi"("User-defined sequence"="User-defined\nsequence") -> ("Sequence Preview"=→"Sequence\npreview":cluster{dbl[], dbl[]}[])
    n102 = call "arduino_data_and_filters_V2_subVI.vi"("loop iteration number"=w244, "arduino 1-6 address and errors"=w320, "arduinos on?"=w252) -> ("arduino 1-6 addresses and errors out"=w319:T32, "arduino 1-6 data out"=w318:T33, "arduinos on? output"=w248:bool)  [unwired: 6 in]
    n103 = call "Elapsed Time2"("Set Start Time (s)"=w261) -> ("Elapsed Time (s)"=w236:dbl)  [unwired: 11 in, 7 out]
    n104 = Fract/Exp String To Number(string=w318) -> (number=w310:T17)  [unwired: 3 in, 1 out]
    n105 = event shown="[5] \"Import sequence file\": Value Change" {
      selector: _ -> [_ _ _ _ _ _]
      dyn-events: _ -> [_ _ _ _ _ _]
      timeout: 50 -> [_ _ _ _ _ _]
      tunnel: "User-defined\nsequence" -> [_ _ _ _ w371 _]
      tunnel: w236 -> [_ _ w367 _ _ _]
      tunnel: w235 -> [w361 _ w368 _ _ _]
      tunnel: [w361 _ w366 _ _ _] -> w234
      event Timeout {
        n106 = event-data() -> ()  [unwired: 1 in, 1 out]
      }
      event "Clear all charts": Value Change {
        (unwired) T34 [] ("History Data")
        w364 = cluster{dbl}[] [] ("History Data")
        w365 = cluster{"Resistance":sgl}[] [] ("History Data")
        w363 = dbl[] [] ("History Data")
        n107 = event-data() -> ()  [unwired: 1 in, 1 out]
        n108 = property on="K-6430 (Ohm)" class="WFChart (strict)"("History Data"=w365) -> ()  [unwired: 2 in, 2 out]
        n109 = property on="arduino qcm 3" class="WFChart (strict)"("History Data"=w363) -> ()  [unwired: 2 in, 2 out]
        n110 = property on="arduino qcm 1" class="WFChart (strict)"("History Data"=w363) -> ()  [unwired: 2 in, 2 out]
        n111 = property on="Waveform Chart" class="WFChart (strict)"("History Data"=w364) -> ()  [unwired: 2 in, 2 out]
        n112 = property on="QCM plot" class="WFChart (strict)"("History Data"=cluster{dbl, "Resistance out":dbl}[] []) -> ()  [unwired: 2 in, 2 out]
        n113 = property on="K-2100 (Ohm)" class="WFChart (strict)"("History Data"=w365) -> ()  [unwired: 2 in, 2 out]
        n114 = property on="arduino qcm 4" class="WFChart (strict)"("History Data"=w363) -> ()  [unwired: 2 in, 2 out]
        n115 = property on="K-2420 (Ohm)" class="WFChart (strict)"("History Data"=w365) -> ()  [unwired: 2 in, 2 out]
        n116 = property on="pressure chart" class="WFChart (strict)"("History Data"=w364) -> ()  [unwired: 2 in, 2 out]
        n117 = property on="arduino qcm 2" class="WFChart (strict)"("History Data"=w363) -> ()  [unwired: 2 in, 2 out]
        n118 = property on="arduino qcm 5" class="WFChart (strict)"("History Data"=w363) -> ()  [unwired: 2 in, 2 out]
      }
      event "Tare elapsed time": Value Change {
        n119 = event-data() -> ()  [unwired: 1 in, 1 out]
        n120 = call "Display Message to User2"() -> ("OK"=w369:bool)  [unwired: 10 in, 1 out]
        n121 = Select(t=w367, s=w369, f=w368) -> (s? t:f=w366:dbl)
      }
      event "Clear sequence": Value Change {
        n122 = event-data() -> ()  [unwired: 1 in, 1 out]
        n123 = property on="User-defined\nsequence" class="Tbl (strict)"("Value"=string[][] []) -> ()  [unwired: 2 in, 2 out]
      }
      event "Save sequence": Value Change {
        n124 = event-data() -> ()  [unwired: 1 in, 1 out]
        n125 = call-poly <vilib>:"Write To Spreadsheet File.vi"("2D data"=w371) -> ()  [unwired: 7 in, 1 out]
      }
      event "Import sequence file": Value Change {
        n126 = event-data() -> ()  [unwired: 1 in, 1 out]
        n127 = call-poly <vilib>:"Read From Spreadsheet File.vi"() -> ("all rows"=w372:string[][])  [unwired: 7 in, 4 out]
        n128 = property on="User-defined\nsequence" class="Tbl (strict)"("Value"=w372) -> ()  [unwired: 2 in, 2 out]
      }
    }
    n129 = Divide(x=w310, y=T17 {"f"=1000000.0, "f"=1000000.0, "f"=1000000.0, "f"=1000000.0, "f"=1000000.0}) -> (x/y=w266:T17)
    n130 = Unbundle(w212) -> ("sequence on?"=w216:bool, "current  step # out"=w215:i32, "sequence end time"=w214:timestamp)
    n131 = case shown="True" w248 {
      tunnel: w266 -> [_ w348]
      frame False {
      }
      frame True {
        "Arduino QCM freq" <- w348
        "Arduino QCM plots" <- w348
      }
    }
    n132 = Unbundle("Data saving options") -> ("Save during sequence only"=w280:bool, "Save now"=w282:bool, "Delay between data points (s)"=w263:dbl, "Experiment Notes"=w264:string)  [unwired: 2 out]
    n133 = Subtract(x=w259, y=w234) -> (x-y=w258:dbl)
    n134 = And(x=w216, y=w280) -> (x .and. y?=w279:bool)
    n135 = Divide(x=w258, y=60.0) -> (x/y=w226:dbl)
    "Elapsed time (min)" <- w226
    n136 = call "data_headers_subVI.vi"("Experiment Notes"=w264, "Sample names"="Sample names") -> ("data headers"=w311:string[])  [unwired: 9 in]
    n137 = Multiply(x=w263, y=u32 1000 ("x")) -> (x*y=w324:dbl)
    n138 = Or(x=w279, y=w282) -> (x .or. y?=w274:bool)
    n139 = Wait (ms)(milliseconds to wait=w324) -> ()  [unwired: 1 out]
    n140 = property on="Currently saving data" class="Bool (strict)"("Value"=w274) -> ()  [unwired: 2 in, 2 out]
    n141 = Get Date/Time In Seconds() -> (seconds since 1Jan1904=w347:timestamp)
    n142 = Number To Engineering String ("elapsed time (min)")(4:w226) -> (0:w231:string)  [unwired: 3 in]
    n143 = Format Date/Time String(time format string (%c)="%Y-%m-%d %H:%M:%S%2u", seconds (now)=w347) -> (date/time string=w321:string)  [unwired: 1 in]
    n144 = Unbundle(w239) -> ("String data out"=w230:string, w229:string, w228:string, w227:string)
    n145 = Unbundle(w317) -> ("String"=w232:string, "String"=w323:string, "String"=w322:string)
    n146 = Unbundle(w222) -> ("String"=w221:string, "String"=w220:string)
    n147 = Unbundle(w308) -> ("pressure"=w307:string, "RH"=w306:string, "gas flow"=w305:string, "vapor flow"=w304:string)
    n148 = Unbundle ("arduino 1-6")(w318) -> ("f"=w316:string, "f"=w315:string, "f"=w314:string, "f"=w313:string, "f"=w312:string)
    n149 = Build Array(w321, w231, w230, w229, w228, w227, w232, w323, w322, w221, w220, w307, w306, w305, w304, w316, w315, w314, w313, w312) -> (w329:string[])
    "State date/time" <- w225
  }
  n150 = Unbundle(w73) -> (w72:bool, "VISA resource name out"=w71:refnum<visa-resource-name>, "error out"=w70:errorcluster)
  n151 = Unbundle(w69) -> ("Boolean"=w68:bool, "VISA out"=w67:refnum<visa-resource-name>, "error out"=w66:errorcluster)
  n152 = call-poly <vilib>:"Write To Spreadsheet File.vi"("1D data"=w25, "file path (dialog if empty)"=w54) -> ("new file path (Not A Path if cancelled)"=w58:path)  [unwired: 6 in]
  n153 = case shown="True" w44 {
    tunnel: w24 -> [_ w435]
    tunnel: [errorcluster {"status"=FALSE, "code"=0, "source"=""} ("error out") w422] -> w6
    frame False {
    }
    frame True {
      n154 = Unbundle(w435) -> ("task out"=w434:refnum<k21>, "error out"=w433:errorcluster, "task out"=w432:refnum<k21>, "error out"=w431:errorcluster, "task out"=w430:refnum<k21>, "error out"=w429:errorcluster, "VISA Refnum out"=w428:refnum<visa-resource-name>, "error out"=w427:errorcluster)
      n155 = disable-structure shown="Disabled" {
        disable-tunnel: [w444 _] -> w426
        disable-tunnel: w434 -> [w443 _]
        disable-tunnel: w433 -> [w442 _]
        frame Disabled {
          n156 = call <vilib>:"DAQmx Stop Task.vi"("task/channels in"=w443, "error in"=w442) -> ("task out"=w445:refnum<k21>, "error out"=w446:errorcluster)  [unwired: 12 in]
          n157 = call <vilib>:"DAQmx Clear Task.vi"("task in"=w445, "error in"=w446) -> ("error out"=w444:errorcluster)  [unwired: 13 in]
        }
        frame Enabled {
        }
      }
      n158 = call <vilib>:"DAQmx Stop Task.vi"("task/channels in"=w432, "error in"=w431) -> ("task out"=w439:refnum<k21>, "error out"=w438:errorcluster)  [unwired: 12 in]
      n159 = call <vilib>:"DAQmx Stop Task.vi"("task/channels in"=w430, "error in"=w429) -> ("task out"=w440:refnum<k21>, "error out"=w441:errorcluster)  [unwired: 12 in]
      n160 = VISA Clear(VISA resource name=w428, error in (no error)=w427) -> (VISA resource name out=w437:refnum<visa-resource-name>, error out=w436:errorcluster)
      n161 = VISA Close(VISA resource name=w437, error in (no error)=w436) -> (error out=w423:errorcluster)
      n162 = call <vilib>:"DAQmx Clear Task.vi"("task in"=w439, "error in"=w438) -> ("error out"=w425:errorcluster)  [unwired: 13 in]
      n163 = call <vilib>:"DAQmx Clear Task.vi"("task in"=w440, "error in"=w441) -> ("error out"=w424:errorcluster)  [unwired: 13 in]
      n164 = Merge Errors(w426, w425, w424, w423) -> (w422:errorcluster)
    }
  }
  n165 = Unbundle(w47) -> (w52:bool, "VISA resource name out"=w51:refnum<visa-resource-name>, "error out"=w50:errorcluster)
  n166 = call "arduino_close_subIV.vi"("arduino 1-6 addresses and errors out"=w27, "arduinos on?"=w26) -> ()  [unwired: 10 in]
  n167 = case shown="True" w15 {
    tunnel: w14 -> [_ w450]
    tunnel: w13 -> [w447 w449]
    tunnel: [w447 w448] -> w12
    frame False {
    }
    frame True {
      n168 = call "Close.vi"("VISA resource name"=w450, "error in (no error)"=w449) -> ("error out"=w448:errorcluster)  [unwired: 17 in]
    }
  }
  n169 = Unbundle(w64) -> ("Boolean"=w63:bool, "VISA resource name out"=w62:refnum<visa-resource-name>, "error out"=w61:errorcluster)
  n170 = case shown="True" w72 {
    tunnel: w71 -> [_ w454]
    tunnel: w70 -> [w451 w453]
    tunnel: [w451 w452] -> w74
    frame False {
    }
    frame True {
      n171 = call "Enable Output.vi"("error in (no error)"=w453, "Enable Output (T: Enable)"=FALSE, "VISA resource name"=w454) -> ("error out"=w455:errorcluster, "VISA resource name out"=w457:refnum<visa-resource-name>)  [unwired: 7 in]
      n172 = call "Close.vi"("error in (no error)"=w455, "VISA resource name"=w457) -> ("error out"=w452:errorcluster)  [unwired: 9 in]
    }
  }
  n173 = case shown="True" w52 {
    tunnel: w51 -> [_ w460]
    tunnel: w50 -> [w458 w459]
    tunnel: [w458 w461] -> w46
    frame False {
    }
    frame True {
      n174 = call "Enable Output.vi"("error in (no error)"=w459, "Enable Output (F:Off)"=FALSE ("Output (F:Off)"), "VISA resource name"=w460) -> ("error out"=w462:errorcluster, "VISA resource name out"=w463:refnum<visa-resource-name>)  [unwired: 7 out]
      n175 = call "Close.vi"("error in (no error)"=w462, "VISA resource name"=w463) -> ("error out"=w461:errorcluster)  [unwired: 9 out]
    }
  }
  n176 = case shown="True" w68 {
    tunnel: w66 -> [w465 w468]
    tunnel: [w465 w467] -> w75
    tunnel: w67 -> [_ w466]
    frame False {
    }
    frame True {
      n177 = call "srsQcm200Close.vi"("error in"=w468, "Visa in"=w466) -> ("error out"=w467:errorcluster)  [unwired: 3 in]
    }
  }
  n178 = call-poly <vilib>:"Write To Spreadsheet File.vi"("append to file? (new file:F)"=TRUE, "2D data"=w30, "file path (dialog if empty)"=w58) -> ()  [unwired: 5 in, 1 out]
  n179 = case shown="True" w63 {
    tunnel: w62 -> [_ w472]
    tunnel: w61 -> [w469 w471]
    tunnel: [w469 w470] -> w60
    frame False {
    }
    frame True {
      n180 = VISA Close(VISA resource name=w472, error in (no error)=w471) -> (error out=w470:errorcluster)
    }
  }
  n181 = call <vilib>:"Simple Error Handler.vi"("error in (no error)"=w6) -> ()  [unwired: 4 in, 5 out]
  n182 = Merge Errors(w46, w60, w74, w12, w75, w5) -> (w81:errorcluster)
  n183 = call <vilib>:"Simple Error Handler.vi"("error in (no error)"=w81) -> ()  [unwired: 4 in, 5 out]
